vi "Examen.vi"() -> ()   [LabVIEW 2020]
panel:
  in  "Operaciones":T1(ring)
  in  "stop":bool
  out "Resultado":dbl
  in  "Dato #2":i32
  in  "Dato #1/Grados":i32
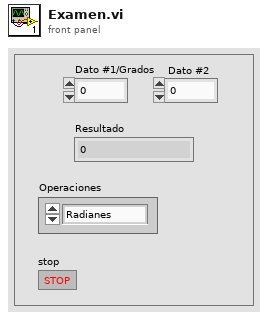
[diagram p1: front panel]
types:
  T1 = enum16{"Radianes", "Tangente", "Coseno", "Seno", "Raiz Cuadrada", "División", "MUltiplicación", "Resta", "Suma"}
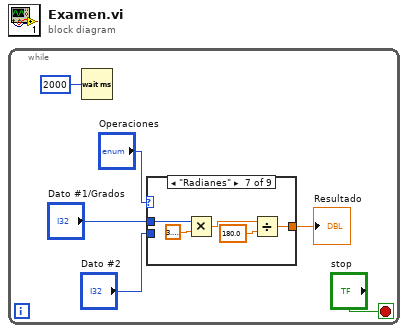
[diagram p0: block diagram]
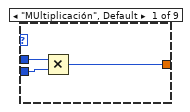
[diagram p2: hidden frame]
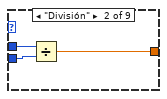
[diagram p3: hidden frame]
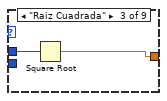
[diagram p4: hidden frame]
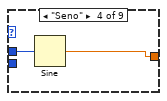
[diagram p5: hidden frame]
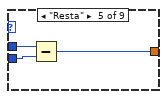
[diagram p6: hidden frame]
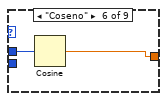
[diagram p7: hidden frame]
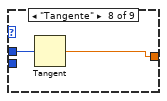
[diagram p8: hidden frame]
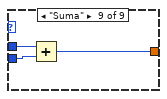
[diagram p9: hidden frame]
diagram:
  n1 = while {
    stop <- "stop" stop-if-true
    n2 = Wait (ms)(milliseconds to wait=u32 2000) -> ()  [unwired: 1 out]
    n3 = case shown="\"Radianes\"" "Operaciones" {
      tunnel: "Dato #1/Grados" -> [w9 w12 w14 w16 w19 w21 w26 w28 w31]
      tunnel: "Dato #2" -> [w8 w11 _ _ w18 _ _ _ w30]
      tunnel: [w7 w10 w13 w15 w17 w20 w22 w27 w29] -> w1
      frame "MUltiplicación", Default {
        n4 = Multiply(x=w9, y=w8) -> (x*y=w7:i32)
      }
      frame "División" {
        n5 = Divide(x=w12, y=w11) -> (x/y=w10:dbl)
      }
      frame "Raiz Cuadrada" {
        n6 = Square Root(x=w14) -> (sqrt(x)=w13:dbl)
      }
      frame "Seno" {
        n7 = Sine(x=w16) -> (sin(x)=w15:dbl)
      }
      frame "Resta" {
        n8 = Subtract(x=w19, y=w18) -> (x-y=w17:i32)
      }
      frame "Coseno" {
        n9 = Cosine(x=w21) -> (cos(x)=w20:dbl)
      }
      frame "Radianes" {
        n10 = Multiply(x=w26, y=3.141592653589793) -> (x*y=w24:dbl)
        n11 = Divide(x=w24, y=180.0) -> (x/y=w22:dbl)
      }
      frame "Tangente" {
        n12 = Tangent(1:w28) -> (0:w27:dbl)
      }
      frame "Suma" {
        n13 = Add(x=w31, y=w30) -> (x+y=w29:i32)
      }
    }
    "Resultado" <- w1
  }
